vi "Execute.vi"(8 "error in (no error)":errorcluster, 11 "Process Model in":refnum<class "Process Model.lvclass">) -> (0 "error out":errorcluster, 3 "Process Model out":refnum<class "Process Model.lvclass">)   [LabVIEW 2017, in "Parallelizer Example.lvlib" / "Process Model.lvclass"]
uses:
  <vilib>/gpm_packages/@cs/test-executive/Source/Sandbox/Parallelizer Example/Process Model/Process Model.lvclass
  C:/Program Files/National Instruments/LabVIEW 2017/vi.lib/ActorFramework/Actor/Actor.lvclass
  <vilib>/gpm_packages/@cs/test-executive/Source/Sandbox/Parallelizer Example/Process Model/Process Model.lvclass/Process Model.ctl
  <vilib>/gpm_packages/@cs/test-executive/Source/Sandbox/Parallelizer Example/iTest Step Messages/Do That Thang Msg/Do That Thang Msg.lvclass/Do That Thang Msg.ctl
  <vilib>/ActorFramework/Message Enqueuer/Message Enqueuer.lvclass/Message Enqueuer.ctl
  <vilib>/ActorFramework/Actor/Actor.lvclass/Actor.ctl
  <vilib>/ActorFramework/Message Enqueuer/Enqueue.vi
  <vilib>/ActorFramework/Message Enqueuer/Init from Existing Queue.vi
  <vilib>/gpm_packages/@cs/test-executive/Source/Sandbox/Parallelizer Example/iTest Step/iTest Step.lvclass
  <vilib>/gpm_packages/@cs/test-executive/Source/Sandbox/Parallelizer Example/iTest Step Messages/Do That Thang Msg/Do That Thang Msg.lvclass
  C:/Program Files/National Instruments/LabVIEW 2017/vi.lib/ActorFramework/Message/Message.lvclass
  <vilib>/ActorFramework/Stop Msg/Stop Msg.lvclass
  <vilib>/ActorFramework/Message Priority Queue/Priority Enqueue.vi
  <vilib>/ActorFramework/Message Enqueuer/Message Enqueuer.lvclass
  <vilib>/gpm_packages/@cs/test-executive/Source/Test Executive/TestExecutive Ref/TestExecutive Ref.lvclass
  <vilib>/ActorFramework/Actor/Actor.lvclass
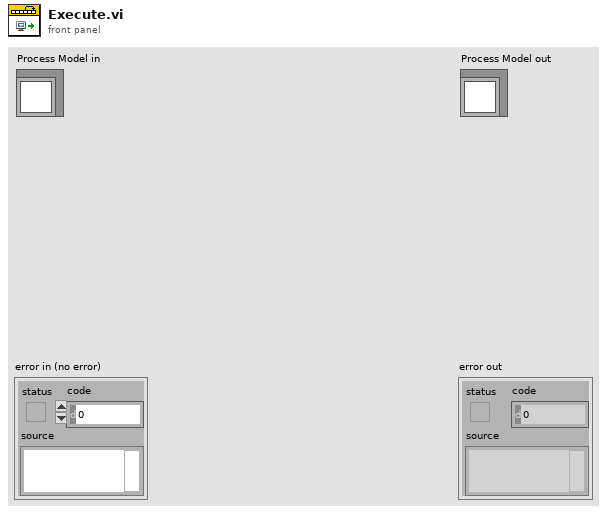
[diagram p1: front panel]
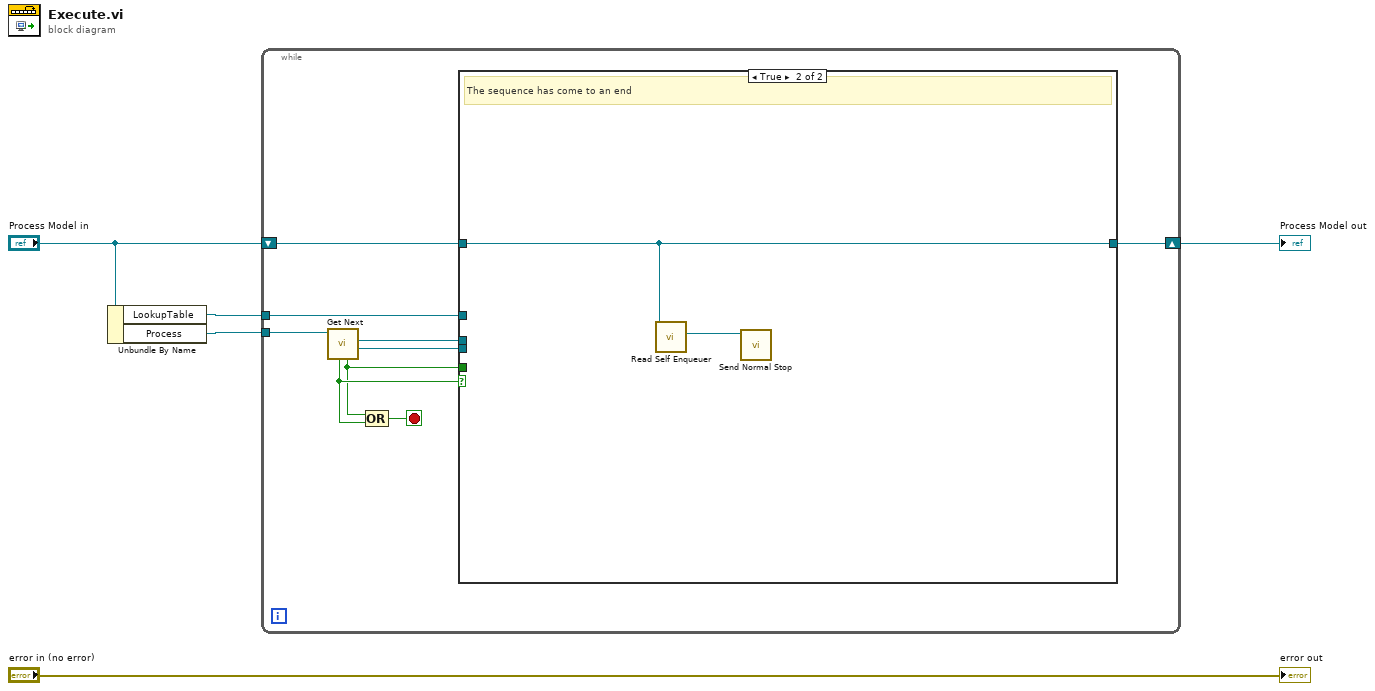
[diagram p0: block diagram]
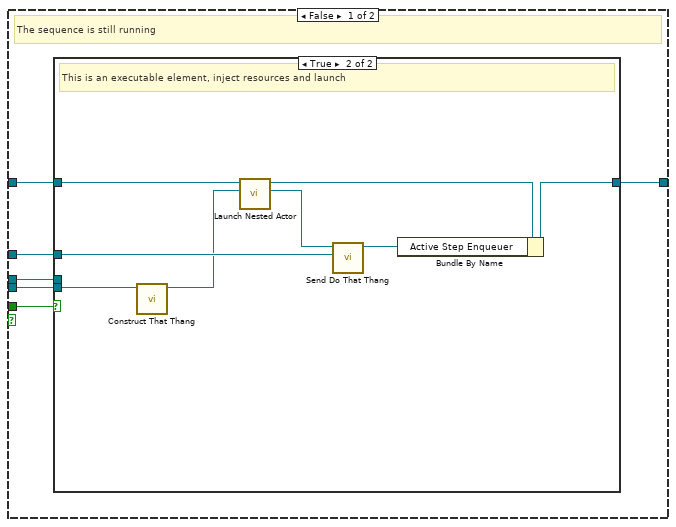
[diagram p2: hidden frame]
diagram:
  n1 = Unbundle By Name("Process Model in") -> ("LookupTable"=w1:refnum<data-value>, "Process"=w2:refnum<data-value>)
  n2 = while {
    shift-right: [w10] -> w3
    shift-left: "Process Model in" -> [w11]
    tunnel: w2 -> [w14]
    tunnel: w1 -> [w6]
    stop <- w13 stop-if-true
    n3 = call <vilib>:"Get Next.vi"("Test Executive Ref"=w14) -> ("Test"=w7:refnum<class "Executioner.lvclass">, "Active Test Executive Ref out"=w8:refnum<data-value>, "Found"=w9:bool, "Complete"=w12:bool)  [unwired: 4 in, 3 out]
    n4 = Compound Arithmetic op=OR(w9, w12) -> (w13:bool)
    n5 = case shown="True" w12 {
      tunnel: [w19 w31] -> w10
      tunnel: w11 -> [w20 w31]
      tunnel: w9 -> [w18 _]
      tunnel: w8 -> [w17 _]
      tunnel: w7 -> [w16 _]
      tunnel: w6 -> [w15 _]
      frame False {
        # "The sequence is still running"
        n6 = case shown="True" w18 {
          tunnel: [w21 w23] -> w19
          tunnel: w20 -> [w21 w29]
          tunnel: w17 -> [_ _]
          tunnel: w16 -> [_ w28]
          tunnel: w15 -> [_ w26]
          frame False {
            # "Not an executable element"
          }
          frame True {
            # "This is an executable element, inject resources and launch"
            n7 = call <vilib>:"Construct That Thang.vi"("Executioner in"=w28) -> ("iTest Step out"=w22:refnum<class "iTest Step.lvclass">)  [unwired: 9 in, 1 out]
            n8 = call <vilib>:"Launch Nested Actor.vi"("Nested Actor"=w22, "Caller Actor in"=w29) -> ("Nested Actor's Enqueuer"=w27:refnum<class "Message Enqueuer.lvclass">, "Caller Actor out"=w24:refnum<class "Process Model.lvclass">)  [unwired: 7 in, 1 out]
            n9 = call <vilib>:"Send Do That Thang.vi"("Lookup Table"=w26, "Message Enqueuer"=w27) -> ("Message Enqueuer out"=w25:refnum<class "Message Enqueuer.lvclass">)  [unwired: 8 in, 1 out]
            n10 = Bundle By Name(cluster=w24, "Active Step Enqueuer"=w25) -> (w23:refnum<class "Process Model.lvclass">)
          }
        }
      }
      frame True {
        # "The sequence has come to an end"
        n11 = call <vilib>:"Read Self Enqueuer.vi"("Actor"=w31) -> ("Self Enqueuer"=w30:refnum<class "Message Enqueuer.lvclass">)  [unwired: 10 in]
        n12 = call <vilib>:"Send Normal Stop.vi"("Message Enqueuer"=w30) -> ()  [unwired: 10 in, 1 out]
      }
    }
  }
  "Process Model out" <- w3
  "error out" <- "error in (no error)"
